vi "步响应index2time.vi"(3 "步响应计算参数 in":T1, 4 "Sampling Rate":dbl=5000.0, 5 "油压1":dbl[](array[numeric]), 6 "行程 in":dbl[](array[numeric])) -> (0 "步响应计算参数 out":T1, 2 "Waveform Graph":cluster{dbl, dbl, dbl[][]}(graph))   [LabVIEW 2013]
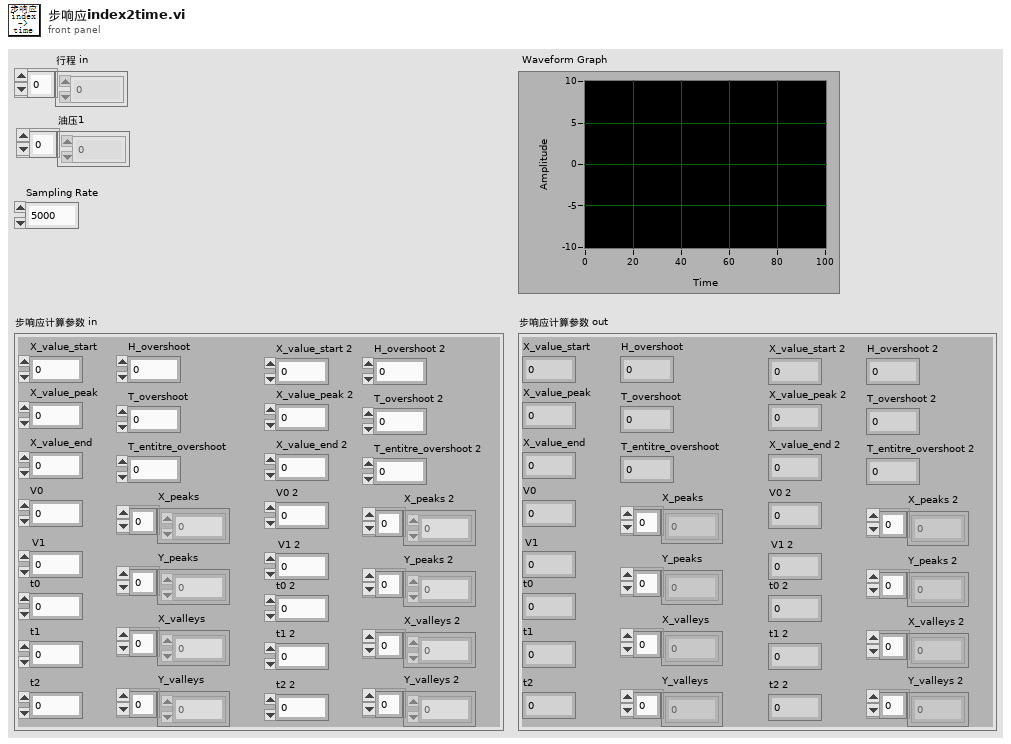
[diagram p1: front panel]
types:
  T1 = cluster{"X_value_start":dbl, "X_value_peak":dbl, "t1":dbl, "X_value_end":dbl, "V0":dbl, "V1":dbl, "t0":dbl, "X_peaks":dbl[], "X_valleys":dbl[], "Y_peaks":dbl[], "Y_valleys":dbl[], "t2":dbl, "H_overshoot":dbl, "T_overshoot":dbl, "T_entitre_overshoot":dbl, "X_value_start 2":dbl, "X_value_peak 2":dbl, "t1 2":dbl, "X_value_end 2":dbl, "V0 2":dbl, "V1 2":dbl, "t0 2":dbl, "X_peaks 2":dbl[], "X_valleys 2":dbl[], "Y_peaks 2":dbl[], "t2 2":dbl, "H_overshoot 2":dbl, "T_overshoot 2":dbl, "T_entitre_overshoot 2":dbl, "Y_valleys 2":dbl[]}
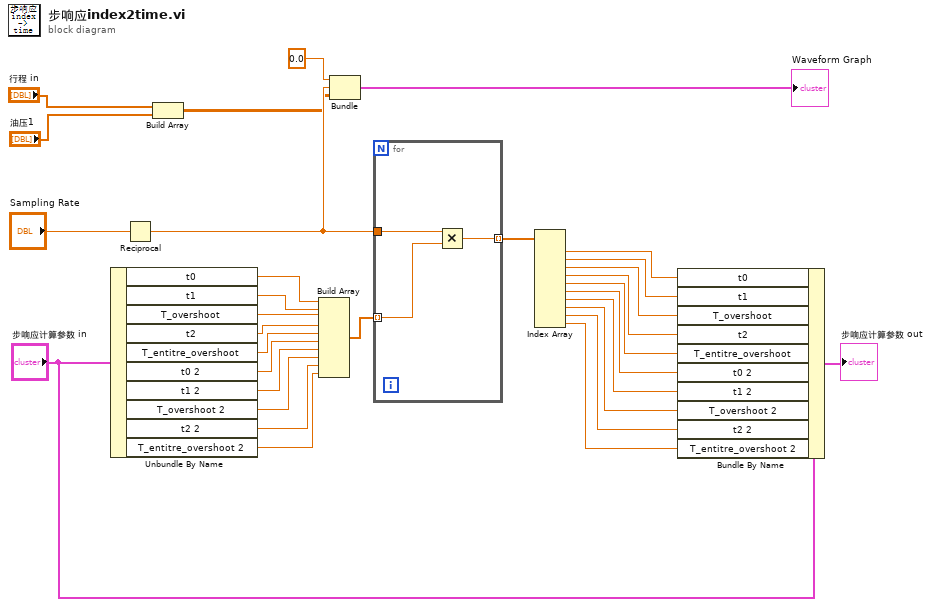
[diagram p0: block diagram]
diagram:
  n1 = Unbundle By Name("步响应计算参数 in") -> ("t0"=w31:dbl, "t1"=w30:dbl, "T_overshoot"=w29:dbl, "t2"=w28:dbl, "T_entitre_overshoot"=w27:dbl, "t0 2"=w13:dbl, "t1 2"=w12:dbl, "T_overshoot 2"=w11:dbl, "t2 2"=w10:dbl, "T_entitre_overshoot 2"=w9:dbl)
  n2 = Reciprocal(x="Sampling Rate") -> (1/x=w14:dbl)
  n3 = Build Array("行程 in", "油压1") -> (w1:dbl[][])
  n4 = Build Array(w31, w30, w29, w28, w27, w13, w12, w11, w10, w9) -> (w25:dbl[])
  n5 = Bundle(0.0, w14, w1) -> (→"Waveform Graph":cluster{dbl, dbl, dbl[][]})  [unwired: 1 in]
  n6 = for {
    tunnel: w14 -> [w34]
    tunnel: w25 -> [w33] mode=indexing
    tunnel: [w32] -> w22 mode=indexing
    n7 = Multiply(x=w34, y=w33) -> (x*y=w32:dbl)
  }
  n8 = Index Array(array=w22) -> (element #1=w21:dbl, element #2=w20:dbl, element #3=w19:dbl, element #4=w18:dbl, element #5=w17:dbl, element #6=w8:dbl, element #7=w7:dbl, element #8=w6:dbl, element #9=w5:dbl, element #10=w4:dbl)  [unwired: 10 in]
  n9 = Bundle By Name(cluster="步响应计算参数 in", "t0"=w21, "t1"=w20, "T_overshoot"=w19, "t2"=w18, "T_entitre_overshoot"=w17, "t0 2"=w8, "t1 2"=w7, "T_overshoot 2"=w6, "t2 2"=w5, "T_entitre_overshoot 2"=w4) -> (→"步响应计算参数 out":T1)
